vi "UDP Rx Main.vi"(8 "error in (no error)":errorcluster, 9 "max size (800)":i32=800, 10 "ports":u16[](array[numeric])=[60000, 60001, 60002, 60003], 11 "Stop Pointer":refnum<class "Pointer.lvclass">) -> (0 "error out":errorcluster)   [LabVIEW 2017]
uses:
  <vilib>/NI/Memory Manager/Classes/Pointer/Pointer.lvclass
  <vilib>/NI/Memory Manager/Classes/Pointer/Pointer.lvclass/Pointer.ctl
  <vilib>/NI/Memory Manager/Classes/Pointer/Write Bool.vi
  <vilib>/NI/Memory Manager/Classes/Pointer/Read I32.vi
  <vilib>/NI/Memory Manager/Classes/Pointer/Read Bool.vi
  <vilib>/NI/Memory Manager/Classes/Pointer/Set Address.vi
  <vilib>/NI/Memory Manager/Classes/Pointer/Set Size.vi
  <vilib>/NI/Memory Manager/Classes/Pointer/Set Internal.vi
  <vilib>/NI/Memory Manager/Classes/Pointer/Write (No Check).vi
  <vilib>/NI/Memory Manager/Classes/Pointer/Write (No Check) Bool.vi
  <vilib>/NI/Memory Manager/Classes/Pointer/Check Move.vi
  <vilib>/NI/Memory Manager/Classes/Pointer/Read (No Check).vi
  <vilib>/NI/Memory Manager/Classes/Pointer/Read (No Check) I32.vi
  <vilib>/NI/Memory Manager/Classes/Pointer/Read (No Check) Bool.vi
  <vilib>/NI/Memory Manager/Classes/Pointer/Get Address.vi
  <vilib>/NI/Memory Manager/Classes/Pointer/Check Null Pointer.vi
  <vilib>/NI/Memory Manager/Classes/Pointer/Check Count.vi
  <vilib>/NI/Memory Manager/Classes/Pointer/Check Bounds (Power of 2).vi
  <vilib>/NI/Memory Manager/Classes/Pointer/Errors.vi
  <vilib>/NI/Memory Manager/Classes/Pointer/Null Pointer.vi
  <vilib>/NI/Memory Manager/Classes/Pointer/Is Null.vi
  <vilib>/NI/Memory Manager/Classes/Pointer/Get Size.vi
  <vilib>/NI/Memory Manager/Classes/Pointer/Out of Bounds.vi
  <vilib>/NI/Memory Manager/Classes/Pointer/Check Bounds.vi
  <vilib>/NI/Memory Manager/Classes/Pointer/Create Error.vi
  <vilib>/NI/Memory Manager/VIs/Source.Write.String.vi
  <vilib>/NI/Memory Manager/Classes/Pointer/Write Pointer Size.vi
  <vilib>/NI/Memory Manager/VIs/Source.Write.Scalar.Base10.vi
  <vilib>/NI/Memory Manager/VIs/Source.Write.Scalar.Base10 (U64).vi
  <vilib>/NI/Memory Manager/Classes/Pointer/Check Pointer Bounds.vi
  <vilib>/NI/Memory Manager/Classes/Pointer/Check Buffer Bounds.vi
  <vilib>/NI/Memory Manager/VIs/New Error Cluster Constant.vi
  <vilib>/NI/Memory Manager/VIs/New Error Cluster Constant (512B).vi
  <vilib>/NI/Memory Manager/VIs/Error Cluster.Set Status.vi
  <vilib>/NI/Memory Manager/VIs/Error Cluster.Set Code.vi
  <vilib>/NI/Memory Manager/VIs/Error Cluster.Set VI Source.vi
  <vilib>/NI/Memory Manager/Constants/Constants.vi
  <vilib>/NI/Memory Manager/Constants/Library Name.vi
  <vilib>/NI/Memory Manager/Classes/Pointer/Pointer Error Info.vi
  <vilib>/NI/Memory Manager/Constants/Pointer Class Name.vi
  <vilib>/NI/Memory Manager/Classes/Pointer/Buffer Underflow.vi
panel:
  out "rx counts":i32[](array[numeric])
  in  "Stop":bool
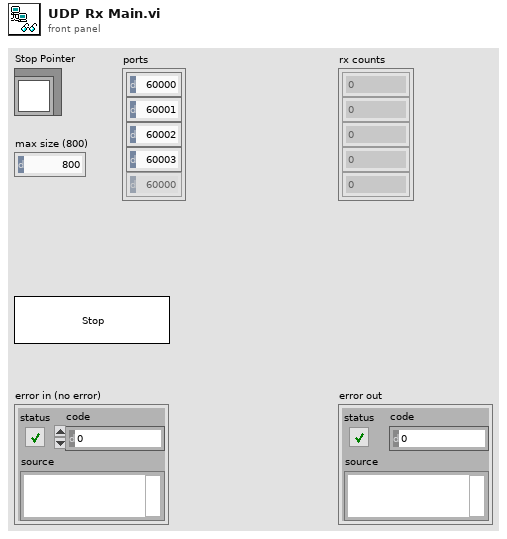
[diagram p1: front panel]
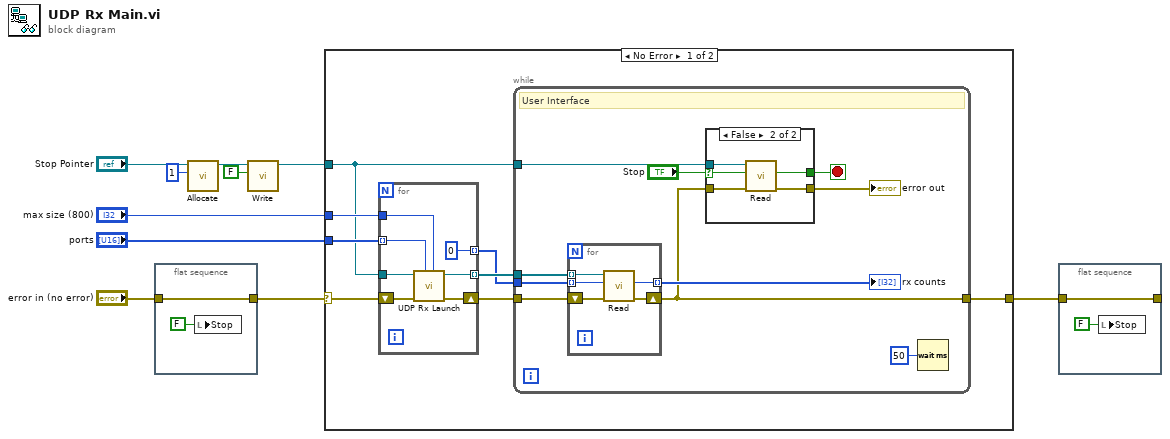
[diagram p0: block diagram]
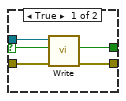
[diagram p2: hidden frame]
diagram:
  n1 = flat-sequence {
    tunnel: "error in (no error)" -> [w12]
    tunnel: [w12] -> w5
    frame #0 {
      n2 = local write "Stop"(FALSE ("Stop")) -> ()
    }
  }
  n3 = call <vilib>:"Allocate.vi"("size"=u64 1, "Pointer in"="Stop Pointer") -> ("Pointer out"=w3:refnum<class "Pointer.lvclass">)  [unwired: 8 in, 1 out]
  n4 = call-poly <vilib>:"Write.vi"("value"=FALSE, "Pointer in"=w3) -> ("Pointer out"=w2:refnum<class "Pointer.lvclass">)  [unwired: 6 in, 3 out]
  n5 = case shown="No Error" w5 {
    selector: w5 -> [w14 w53]
    tunnel: "ports" -> [w20 _]
    tunnel: "max size (800)" -> [w19 _]
    tunnel: w2 -> [w16 _]
    tunnel: [w15 w53] -> w6
    frame No Error {
      n6 = for {
        tunnel: w16 -> [w22]
        tunnel: w20 -> [w25] mode=indexing
        tunnel: w19 -> [w24]
        shift-right: [w27] -> w18
        shift-left: w14 -> [w26]
        tunnel: [w23] -> w17 mode=indexing
        tunnel: [0] -> w13 mode=indexing
        n7 = call "UDP Rx Launch.vi"("max size (548)"=w24, "port"=w25, "error in (no error)"=w26, "Stop Pointer"=w22) -> ("error out"=w27:errorcluster, "Count Pointer"=w23:refnum<class "Pointer.lvclass">)  [unwired: 6 in]
      }
      n8 = while {
        tunnel: w18 -> [w36]
        tunnel: w17 -> [w37]
        tunnel: w16 -> [w35]
        tunnel: [w29] -> w15
        tunnel: w13 -> [w28]
        stop <- w34 stop-if-true
        # "User Interface"
        n9 = for {
          tunnel: w37 -> [w52] mode=indexing
          tunnel: [w49] -> w31 mode=indexing
          shift-right: [w50] -> w29
          shift-left: w36 -> [w51]
          tunnel: w28 -> [w48] mode=indexing
          n10 = call-poly <vilib>:"Read.vi"("error in (no error)"=w51, "value in"=w48, "Pointer in"=w52) -> ("error out"=w50:errorcluster, "value out"=w49:i32)  [unwired: 5 in, 2 out]
        }
        "rx counts" <- w31
        n11 = case shown="False" "Stop" {
          selector: "Stop" -> [w38 w43]
          tunnel: w35 -> [w42 w47]
          tunnel: w29 -> [w41 w46]
          tunnel: [w40 w45] -> w34
          tunnel: [w39 w44] -> w32
          frame True {
            n12 = call-poly <vilib>:"Write.vi"("error in (no error)"=w41, "value"=w38, "Pointer in"=w42) -> ("error out"=w39:errorcluster, "value"=w40:bool)  [unwired: 5 in, 2 out]
          }
          frame False {
            n13 = call-poly <vilib>:"Read.vi"("error in (no error)"=w46, "value in"=w43, "Pointer in"=w47) -> ("error out"=w44:errorcluster, "value out"=w45:bool)  [unwired: 5 in, 2 out]
          }
        }
        "error out" <- w32
        n14 = Wait (ms)(milliseconds to wait=u32 50) -> ()  [unwired: 1 out]
      }
    }
    frame Error {
    }
  }
  n15 = flat-sequence {
    tunnel: w6 -> [w55]
    tunnel: [w55] -> _
    frame #0 {
      n16 = local write "Stop"(FALSE ("Stop")) -> ()
    }
  }
